vi "Connect servo.vi"(8 "error in (no error)":errorcluster, 10 "IP address":string, 11 "Connection in":variant) -> (0 "error out":errorcluster, 2 "Is connected":bool, 3 "Connection out":variant)   [LabVIEW 2017, in "Servo drive module.lvlib"]
doc: "Connect to physical controller with a given IP address, if is not alredy connected.\nparams:\nconnection - (variant)\nIP address - (string)\nreturns:\nConnection (variant)\nIs connected (boolean)"
uses:
  Servo drive module.lvlib
  <vilib>/addons/eal4LabVIEW/ApiLib/Connection control/ealApiConnect_string_UInt32.vi
  <vilib>/addons/eal4LabVIEW/eal4LabVIEW.lvlib
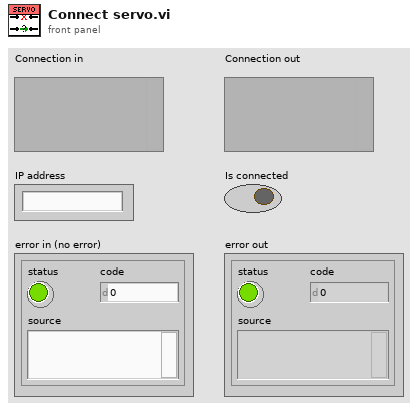
[diagram p1: front panel]
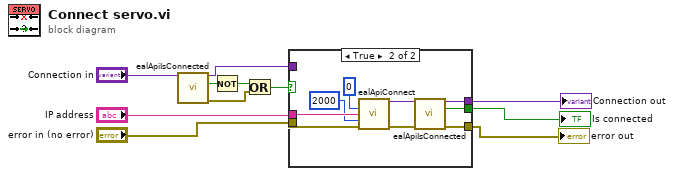
[diagram p0: block diagram]
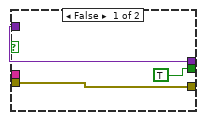
[diagram p2: hidden frame]
diagram:
  n1 = call <vilib>:"ealApiIsConnected.vi"("connection in"="Connection in") -> ("connection out"=w1:variant, "is connected"=w3:bool, "error out"=w6:errorcluster)  [unwired: 12 in]
  n2 = Not(x=w3) -> (.not. x?=w5:bool)
  n3 = Or(x=w5, y=w6) -> (x .or. y?=w4:bool)
  n4 = case shown="True" w4 {
    tunnel: w1 -> [w14 _]
    tunnel: "IP address" -> [_ w23]
    tunnel: [w14 w19] -> w8
    tunnel: [w12 w16] -> w10
    tunnel: "error in (no error)" -> [w12 w15]
    tunnel: [TRUE w18] -> w9
    frame False {
    }
    frame True {
      n5 = call-poly <vilib>:"ealApiConnect.vi"("maximum no of axes"=0, "ip address"=w23, "leaseTimeout"=u32 2000, "error in (no error)"=w15) -> ("connection out"=w20:variant, "error out"=w17:errorcluster)  [unwired: 10 in]
      n6 = call <vilib>:"ealApiIsConnected.vi"("connection in"=w20, "error in (no error)"=w17) -> ("connection out"=w19:variant, "is connected"=w18:bool, "error out"=w16:errorcluster)  [unwired: 11 in]
    }
  }
  "error out" <- w10
  "Is connected" <- w9
  "Connection out" <- w8
